vi "RecrystalliseAHK.vi"(7 "ControllerSettingsRef":refnum<vi>, 8 "error in (no error)":errorcluster, 11 "XAOMsetting":refnum<vi>) -> (0 "error out":errorcluster)   [LabVIEW 2019]
uses:
  controls/xAOMSettings/XAOMsetting.xctl
  controls/ControllerSettings.ctl
  controls/GlobalExp.vi
  Global.lvlib
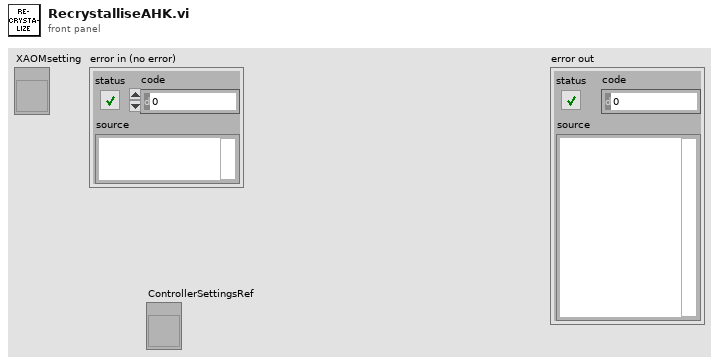
[diagram p1: front panel]
types:
  T1 = typedef "ControllerSettings.ctl" = cluster{"Aux Sequence":bool, "Camera":bool, "Recrystallize":bool, "Raw graph":bool, "Mean graph":bool, "Calculate probs":bool, "Find fit":bool, "ReX Time [s] :":dbl, "Lock Voltage :":dbl, "Line trig ":bool, "Check Fluo":bool, "Pre Sequence":bool}
  T2 = cluster{"HighPowerNum":dbl, "LowPowerNum":dbl, "PIDnum":dbl, "DeltaFreq":dbl, "BaseFreq":dbl, "AOMout":dbl, "ButtonSelected":enum16{"PID", "Low", "High"}, "AO3":bool}
  T3 = typedef "MasterExpControl.ctl" = cluster{"Main Steps":dbl, "Main Runs":dbl, "ExpStatus":enum16{"Innit", "Stop", "Idle", "MainRunning", "AuxRunning"}, "Main Current Step":dbl, "ExpNum":dbl, "NewData":bool, "date":string, "command":string, "Stop":bool, "Pause":bool, "Mathematica":string, "Main/Meta":bool, "UpdateMath":bool, "Camera":bool, "MetaExpOver":bool, "NextMetaExp":bool}
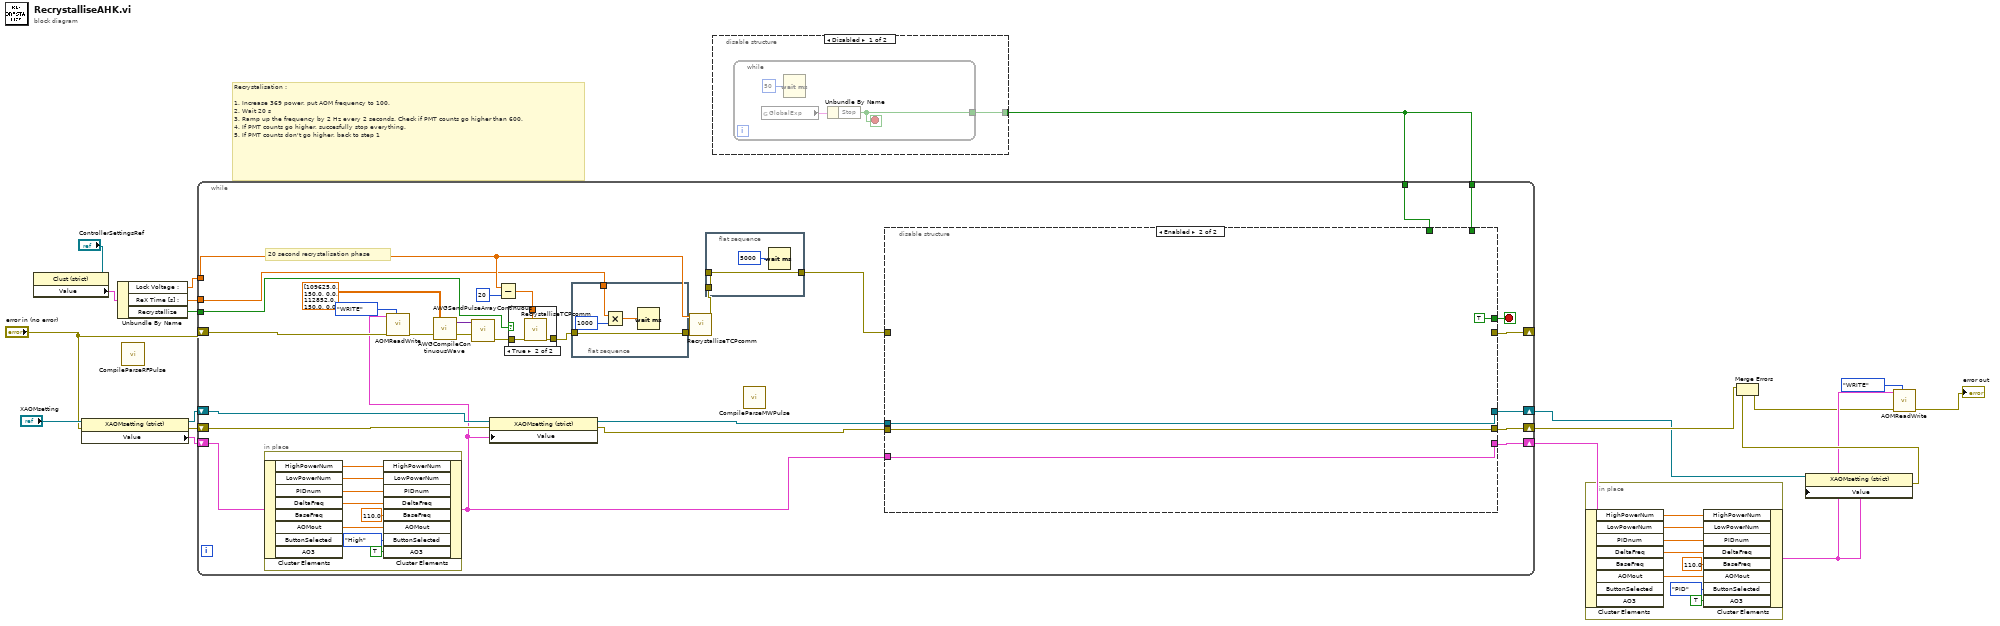
[diagram p0: block diagram]
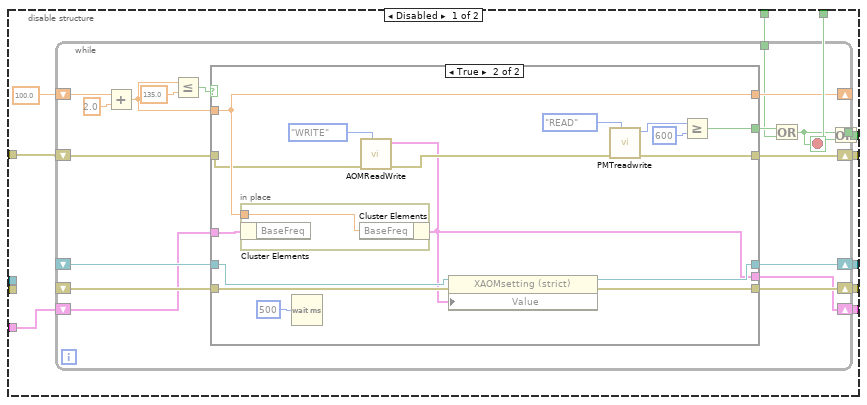
[diagram p4: hidden frame]
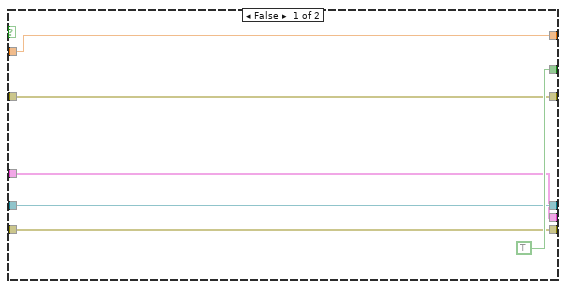
[diagram p5: hidden frame]
diagram:
  # "Recrystalisation :\n\n1. Increase 369 power, put AOM frequency to 100.\n2. Wait 20 s\n3. Ramp up the frequency by 2 Hz every 2 seconds. Check if PMT counts go higher than 600.\n4. If PMT counts go higher, succesfully stop everything.\n5. If PMT counts don't go higher, back to step 1"
  n1 = property class="Clust (strict)"(reference="ControllerSettingsRef") -> ("Value"=w4:T1)  [unwired: 1 in, 2 out]
  n2 = property class="XAOMsetting (strict)"(reference="XAOMsetting", error in="error in (no error)") -> (reference out=w18:refnum<vi>, error out=w16:errorcluster, "Value"=w17:T2)
  n3 = Unbundle By Name(w4) -> ("Lock Voltage :"=w3:dbl, "ReX Time [s] :"=w2:dbl, "Recrystallize"=w1:bool)
  n4 = call "CompileParseRFPulse.vi"() -> ()  [unwired: 2 in, 1 out]
  n5 = disable-structure shown="Disabled" {
    disable-tunnel: [w20 _] -> w14
    frame Disabled {
      n6 = while {
        tunnel: [w21] -> w20
        stop <- w21 stop-if-true
        n7 = global read "GlobalExp.vi" "GlobalExp"() -> (w23:T3)
        n8 = Wait (ms)(milliseconds to wait=u32 50) -> ()  [unwired: 1 out]
        n9 = Unbundle By Name(w23) -> ("Stop"=w21:bool)
      }
    }
    frame Enabled {
    }
  }
  n10 = while {
    shift-right: [w37] -> w12
    shift-left: w18 -> [w51]
    shift-right: [w48] -> w13
    shift-left: w17 -> [w52]
    shift-right: [w49] -> w15
    shift-left: w16 -> [w50]
    shift-right: [w47] -> _
    shift-left: "error in (no error)" -> [w38]
    tunnel: w14 -> [w41]
    tunnel: w14 -> [w40]
    tunnel: w3 -> [w26]
    tunnel: w2 -> [w25]
    tunnel: w1 -> [w24]
    stop <- w46 stop-if-true
    # "20 second recrystalisation phase"
    n11 = in-place {
      n12 = in-place-cluster #1(w52) -> ("HighPowerNum"=w116:dbl, "LowPowerNum"=w115:dbl, "PIDnum"=w114:dbl, "DeltaFreq"=w121:dbl, "AOMout"=w119:dbl)  [unwired: 3 out]
      n13 = in-place-cluster #1("HighPowerNum"=w116, "LowPowerNum"=w115, "PIDnum"=w114, "DeltaFreq"=w121, "BaseFreq"=110.0, "AOMout"=w119, "ButtonSelected"=enum16{"PID", "Low", "High"}."High", "AO3"=TRUE) -> (w32:T2)
    }
    n14 = call "AOMReadWrite.vi"("Enum"=enum16{"READ", "WRITE"}."WRITE", "error in"=w38, "XAOMsetting"=w32) -> ("error out"=w31:errorcluster)  [unwired: 6 in, 2 out]
    n15 = call "AWGCompileContinuousWave.vi"("error in"=w31, "ArbitraryWaveListMW"=dbl[][] [[109625.0, 150.0, 0.0], [112852.0, 150.0, 0.0], [90389.0, 150.0, 0.0], [87173.0, 150.0, 0.0]] ("ArbitraryWaveList")) -> ("error out"=w27:errorcluster, "array MW and RF"=w29:variant[])
    n16 = call "AWGSendPulseArrayContinuous.vi"("error in (no error)"=w27, "AWG pulses array"=w29) -> ("error out"=w30:errorcluster)  [unwired: 8 in, 1 out]
    n17 = property class="XAOMsetting (strict)"(reference=w51, error in=w50, "Value"=w32) -> (reference out=w34:refnum<vi>, error out=w35:errorcluster)
    n18 = Subtract(x=w26, y=20) -> (x-y=w43:dbl)
    n19 = case shown="True" w24 {
      tunnel: [w53 w56] -> w45
      tunnel: w43 -> [_ w55]
      tunnel: w30 -> [w53 w54]
      frame False {
      }
      frame True {
        n20 = call "RecrystalliseTCPcomm.vi"("error in (no error)"=w54, "DC voltage in"=w55) -> ("error out"=w56:errorcluster)  [unwired: 9 in]
      }
    }
    n21 = flat-sequence {
      tunnel: [w125] -> w44
      tunnel: w45 -> [w125]
      tunnel: w25 -> [w122]
      frame #0 {
        n22 = Multiply(x=w122, y=u32 1000) -> (x*y=w124:dbl)
        n23 = Wait (ms)(milliseconds to wait=w124) -> ()  [unwired: 1 out]
      }
    }
    n24 = call "RecrystalliseTCPcomm.vi"("error in (no error)"=w44, "DC voltage in"=w26) -> ("error out"=w36:errorcluster)  [unwired: 9 in]
    n25 = flat-sequence {
      tunnel: [w57] -> w33
      tunnel: [w57] -> _
      tunnel: w36 -> [w57]
      frame #0 {
        n26 = Wait (ms)(milliseconds to wait=u32 5000) -> ()  [unwired: 1 out]
      }
    }
    n27 = call "CompileParseMWPulse.vi"() -> ()  [unwired: 1 in, 1 out]
    n28 = disable-structure shown="Enabled" {
      disable-tunnel: [w68 w111] -> w49
      disable-tunnel: [w67 w110] -> w48
      disable-tunnel: [w66 _] -> w47
      disable-tunnel: [w65 TRUE] -> w46
      disable-tunnel: w41 -> [w63 _]
      disable-tunnel: w40 -> [w62 _]
      disable-tunnel: [w61 w112] -> w37
      disable-tunnel: w33 -> [w60 _]
      disable-tunnel: w32 -> [w59 w110]
      disable-tunnel: w34 -> [_ w112]
      disable-tunnel: w35 -> [_ w111]
      frame Disabled {
        n29 = while {
          shift-right: [w80] -> w66
          shift-left: w60 -> [w84]
          shift-right: [w79] -> _
          shift-left: 100.0 -> [w86]
          tunnel: [w72] -> w64
          shift-right: [w78] -> w61
          shift-left: _ -> [w76]
          shift-right: [w77] -> w68
          shift-left: _ -> [w75]
          shift-right: [w74] -> w67
          shift-left: w59 -> [w70]
          tunnel: w62 -> [w71]
          stop <- w72 stop-if-true
          n30 = Add(x=w86, y=2.0) -> (x+y=w82:dbl)
          n31 = Less Or Equal?(x=w82, y=135.0) -> (x <= y?=w83:bool)
          n32 = case shown="True" w83 {
            tunnel: w84 -> [w91 w95]
            tunnel: w82 -> [w90 w104]
            tunnel: [TRUE w98] -> w73
            tunnel: [w91 w105] -> w80
            tunnel: [w90 w104] -> w79
            tunnel: [w89 w103] -> w78
            tunnel: [w88 w102] -> w77
            tunnel: w76 -> [w89 w101]
            tunnel: w75 -> [w88 w100]
            tunnel: [w87 w93] -> w74
            tunnel: w70 -> [w87 w97]
            frame False {
            }
            frame True {
              n33 = in-place {
                in-place-border: w104 -> [w109]
                n34 = in-place-cluster #2(w97) -> ()  [unwired: 1 out]
                n35 = in-place-cluster #2("BaseFreq"=w109) -> (w93:T2)
              }
              n36 = Wait (ms)(milliseconds to wait=u32 500) -> ()  [unwired: 1 out]
              n37 = call "AOMReadWrite.vi"("Enum"=enum16{"READ", "WRITE"}."WRITE", "error in"=w95, "XAOMsetting"=w93) -> ("error out"=w94:errorcluster)  [unwired: 6 in, 2 out]
              n38 = property class="XAOMsetting (strict)"(reference=w101, error in=w100, "Value"=w93) -> (reference out=w103:refnum<vi>, error out=w102:errorcluster)
              n39 = call "PMTreadwrite.vi"("Enum"=enum16{"READ", "WRITE"}."READ", "error in"=w94) -> ("error out"=w105:errorcluster, "Count Chart"=w107:u32)  [unwired: 8 in]
              n40 = Greater Or Equal?(x=w107, y=u32 600) -> (x >= y?=w98:bool)
            }
          }
          n41 = Or(x=w73, y=w71) -> (x .or. y?=w72:bool)
        }
        n42 = Or(x=w64, y=w63) -> (x .or. y?=w65:bool)
      }
      frame Enabled {
      }
    }
  }
  n43 = in-place {
    n44 = in-place-cluster #3(w13) -> ("HighPowerNum"=w128:dbl, "LowPowerNum"=w127:dbl, "PIDnum"=w126:dbl, "DeltaFreq"=w133:dbl, "AOMout"=w131:dbl)  [unwired: 3 out]
    n45 = in-place-cluster #3("HighPowerNum"=w128, "LowPowerNum"=w127, "PIDnum"=w126, "DeltaFreq"=w133, "BaseFreq"=110.0, "AOMout"=w131, "ButtonSelected"=enum16{"PID", "Low", "High"}."PID", "AO3"=TRUE) -> (w8:T2)
  }
  n46 = property class="XAOMsetting (strict)"(reference=w12, "Value"=w8) -> (error out=w11:errorcluster)  [unwired: 1 in, 1 out]
  n47 = Merge Errors(w15, w11) -> (w6:errorcluster)
  n48 = call "AOMReadWrite.vi"("Enum"=enum16{"READ", "WRITE"}."WRITE", "error in"=w6, "XAOMsetting"=w8) -> ("error out"=→"error out":errorcluster)  [unwired: 6 in, 2 out]
